vi "sub_Channel_Impairments.vi"(7 "Impairments in":T3={"Delay (samples)"=9, "Eb/N0 (10 dB)"=10.0} {"Eb/N0 (10 dB)" format="%.2f"}, 8 "error in (no error)":errorcluster, 10 "QPSK System Parameters":T1={"Samples per Symbol"=8, "symbol map"=[], "Differential PSK"=enum."disable", "PSK type"=0, "M-PSK"=4} {"PSK type" items=["normal", "shifted", "offset"]; "symbol map" format="%.3f"}, 11 "input complex waveform":T2={"t0"=0.0, "dt"=1.0, "Y"=[]} {"Y" format="%.3f"; "dt" format="%^.2e"; "t0" format="%.4f"}) -> (0 "error out":errorcluster, 3 "output cluster":T2={"t0"=0.0, "dt"=1.0, "Y"=[]} caption="Output Complex Waveform" {"Y" format="%.3f"; "dt" format="%^.2e"; "t0" format="%.4f"})   [LabVIEW 2014]
uses:
  <vilib>/addons/Modulation/Analog/controls/Complex Data Waveform.ctl
  <vilib>/addons/Modulation/Digital/Support/Common/Validators/mod_AWGN Validate.vi
  <vilib>/addons/Modulation/Analog/support/mod_Set Error Source.vi
  <vilib>/addons/Modulation/Digital/Impairments/subVIs/mod_createSeeds.vi
  <vilib>/addons/Modulation/Digital/Support/Common/Validators/mod_Validate Samples Per Symbol.vi
  <vilib>/addons/Modulation/Analog/support/Validators/mod_Validate Complex Waveform.vi
  <vilib>/addons/Modulation/Analog/support/Validators/mod_WFErrorHandler.vi
  <vilib>/addons/Modulation/Digital/General/subVIs/mod_Generate Bits PN Sequence.vi
  <vilib>/Analysis/1siggen.llb/Gaussian White Noise (obs 90).vi
  <vilib>/addons/Modulation/niDMT.lvlib
  <vilib>/addons/Modulation/niAMT.lvlib
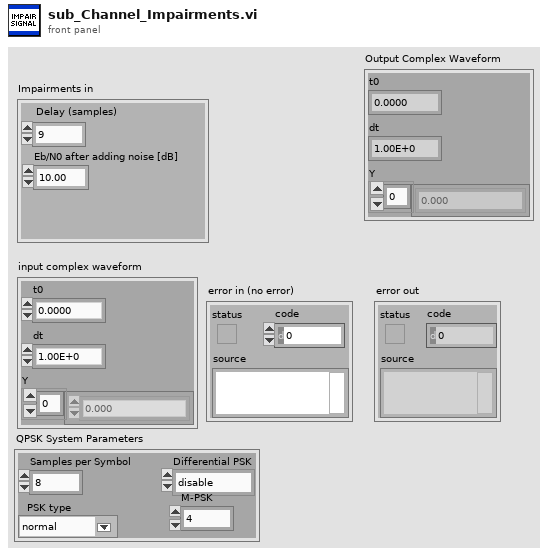
[diagram p1: front panel]
types:
  T1 = cluster{"Samples per Symbol":i32, "symbol map":cdb[], "Differential PSK":enum16{"disable", "enable"}, "PSK type":u16, "M-PSK":i32}
  T2 = typedef "niAMT.lvlib/Complex Data Waveform.ctl" = cluster{"t0":dbl, "dt":dbl, "Y":cdb[]}
  T3 = cluster{"Delay (samples)":i32, "Eb/N0 (10 dB)":dbl}
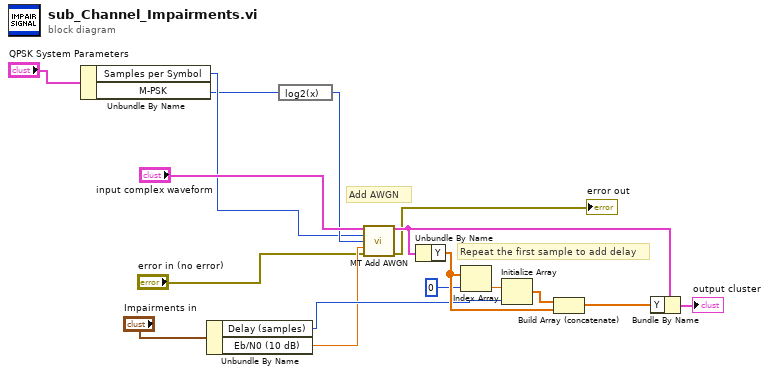
[diagram p0: block diagram]
diagram:
  # "Add AWGN"
  # "Repeat the first sample to add delay"
  n1 = Unbundle By Name("QPSK System Parameters") -> ("Samples per Symbol"=w3:i32, "M-PSK"=w1:i32)
  n2 = Unbundle By Name("Impairments in") -> ("Delay (samples)"=w9:i32, "Eb/N0 (10 dB)"=w8:dbl)
  n3 = expression code="log2(x)"(w1) -> (w4:i32)
  n4 = call <vilib>:"MT Add AWGN.vi"("input complex waveform"="input complex waveform", "samples per symbol (16)"=w3, "bits per symbol (1)"=w4, "Eb/N0 (10 dB)"=w8, "error in (no error)"="error in (no error)") -> ("output complex waveform"=w16:T2, "error out"=→"error out":errorcluster)  [unwired: 8 in, 1 out]
  n5 = Unbundle By Name(w16) -> ("Y"=w13:cdb[])
  n6 = Index Array(array=w13, index=0) -> (element=w11:cdb)
  n7 = Initialize Array(w11, w9) -> (w12:cdb[])
  n8 = Build Array (concatenate)(w12, w13) -> (w17:cdb[])
  n9 = Bundle By Name(cluster=w16, "Y"=w17) -> (→"output cluster":T2)
